vi "crc(SubVI).vi"(11 "String":string) -> (3 "CRC-16 MODBUS Byte Swap 2":string)   [LabVIEW 2020]
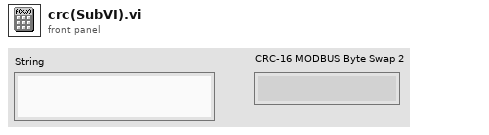
[diagram p1: front panel]
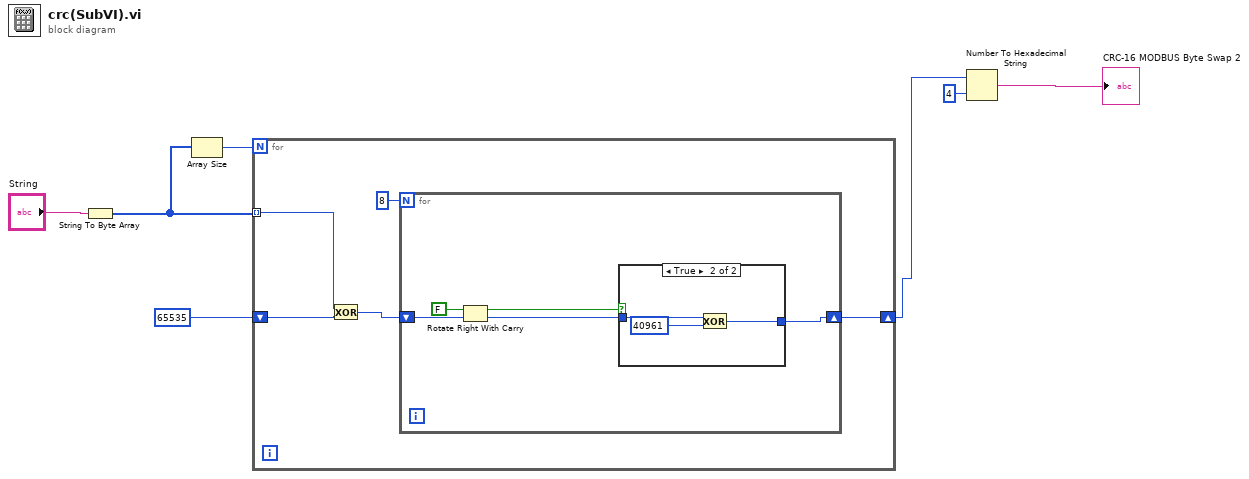
[diagram p0: block diagram]
diagram:
  n1 = String To Byte Array(string="String") -> (unsigned byte array=w4:u8[])
  n2 = Array Size(array=w4) -> (size(s)=w3:i32)
  n3 = for {
    N: w3 -> [_]
    tunnel: w4 -> [w12] mode=indexing
    shift-right: [w10] -> w7
    shift-left: u16 65535 -> [w9]
    n4 = Exclusive Or(1:w9, 2:w12) -> (0:w11:u16)
    n5 = for {
      N: 8 -> [_]
      shift-right: [w13] -> w10
      shift-left: w11 -> [w17]
      n6 = Rotate Right With Carry(2:w17, 3:FALSE ("carry")) -> (0:w14:u16, 1:w15:bool)
      n7 = case shown="True" w15 {
        tunnel: w14 -> [w18 w21]
        tunnel: [w18 w19] -> w13
        frame False {
        }
        frame True {
          n8 = Exclusive Or(1:u16 40961 ("y"), 2:w21) -> (0:w19:u16)
        }
      }
    }
  }
  n9 = Number To Hexadecimal String(1:i16 4 ("width (-)"), 2:w7) -> (0:→"CRC-16 MODBUS Byte Swap 2":string)
